vi "Start Acquisition.vi"(8 "error in (no error)":errorcluster, 11 "CCDCamera in":refnum<class "Real Camera.lvclass">) -> (0 "error out":errorcluster, 3 "CCDCamera out":refnum<class "Real Camera.lvclass">)   [LabVIEW 2018, in "Real Camera.lvclass"]
doc: "Start an acquisition"
uses:
  Real Camera.lvclass
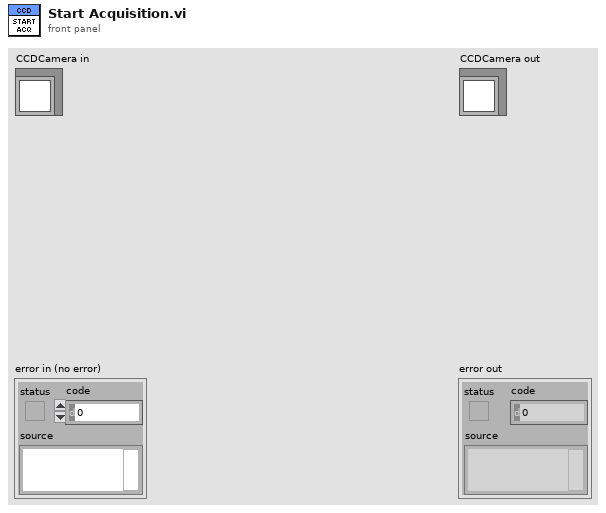
[diagram p1: front panel]
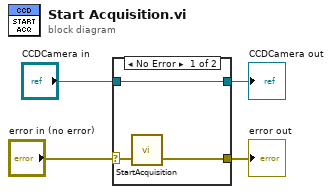
[diagram p0: block diagram]
diagram:
  n1 = case shown="No Error" "error in (no error)" {
    selector: "error in (no error)" -> [w7 w9]
    tunnel: [w5 w9] -> w3
    tunnel: [w6 w8] -> w1
    tunnel: "CCDCamera in" -> [w6 w8]
    frame No Error {
      n2 = call <userlib>:"StartAcquisition.vi"("error in (no error)"=w7) -> ("error out"=w5:errorcluster)  [unwired: 1 in, 1 out]
    }
    frame Error {
    }
  }
  "error out" <- w3
  "CCDCamera out" <- w1
